vi "Tree.vi"   [LabVIEW 2016]
uses:
  subVIs/Add XY (single).vi
  subVIs/Add float (single).vi
  subVIs/Subtract float (single).vi
  subVIs/Multiply float (single).vi
  subVIs/Divide float (single).vi
  subVIs/Sort Ascending (multiple).vi
  subVIs/Decimate (multiple).vi
  subVIs/Add float (multiple).vi
  subVIs/Subtract float (multiple).vi
  subVIs/Multiply float (multiple).vi
  subVIs/Divide float (multiple).vi
  <vilib>/measure/maresamp.llb/Resample N Pairs of Arrays (single shot).vi
  subVIs/Derivative (multiple).vi
  subVIs/Derivative (single).vi
  subVIs/Sort Ascending (single).vi
  subVIs/Decimate (single).vi
  xy_utilities.lvlib
  <vilib>/measure/NI_MAPro.lvlib
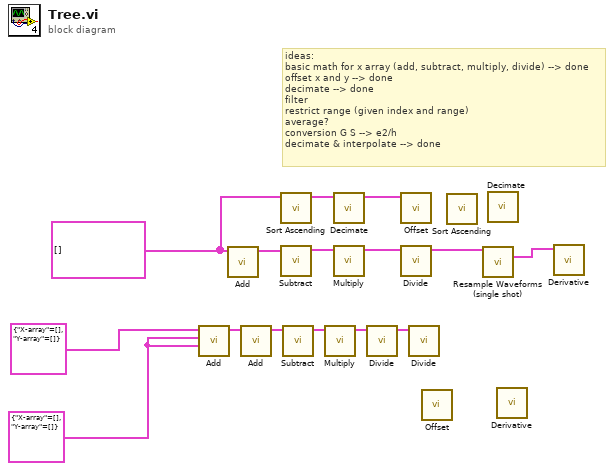
[diagram p0: block diagram]
diagram:
  w8 = cluster{"X-array":dbl[], "Y-array":dbl[]}[] [] ("Multiple XY-data in")
  w10 = cluster{"X-array":dbl[], "Y-array":dbl[]} {"X-array"=[], "Y-array"=[]} ("XY-data in")
  # "ideas:\nbasic math for x array (add, subtract, multiply, divide) --> done\noffset x and y --> done\ndecimate --> done\nfilter\nrestrict range (given index and range)\naverage?\nconversion G S --> e2/h\ndecimate & interpolate --> done"
  n1 = call-poly "Add.vi"("y XY-data in"=w10, "x XY-data in"=w10, "XY-data in"=cluster{"X-array":dbl[], "Y-array":dbl[]} {"X-array"=[], "Y-array"=[]}) -> ("XY-data out"=w5:cluster{"X-array":dbl[], "Y-array":dbl[]})  [unwired: 7 in, 1 out]
  n2 = call-poly "Add.vi"("Multiple XY-data in"=w8) -> ("Multiple XY-data out"=w13:cluster{"X-array":dbl[], "Y-array":dbl[]}[])  [unwired: 9 in, 1 out]
  n3 = call-poly "Add.vi"("XY-data in"=w5) -> ("XY-data out"=w4:cluster{"X-array":dbl[], "Y-array":dbl[]})  [unwired: 9 in, 1 out]
  n4 = call-poly "Sort Ascending.vi"("Multiple XY-data in"=w8) -> ("Multiple XY-data out"=w7:cluster{"X-array":dbl[], "Y-array":dbl[]}[])  [unwired: 9 in, 1 out]
  n5 = call-poly "Subtract.vi"("Multiple XY-data in"=w13) -> ("Multiple XY-data out"=w15:cluster{"X-array":dbl[], "Y-array":dbl[]}[])  [unwired: 9 in, 1 out]
  n6 = call-poly "Subtract.vi"("XY-data in"=w4) -> ("XY-data out"=w3:cluster{"X-array":dbl[], "Y-array":dbl[]})  [unwired: 9 in, 1 out]
  n7 = call-poly "Multiply.vi"("XY-data in"=w3) -> ("XY-data out"=w2:cluster{"X-array":dbl[], "Y-array":dbl[]})  [unwired: 9 in, 1 out]
  n8 = call-poly "Decimate.vi"("Multiple XY-data in"=w7) -> ("Multiple XY-data out"=w9:cluster{"X-array":dbl[], "Y-array":dbl[]}[])  [unwired: 9 in, 1 out]
  n9 = call-poly "Multiply.vi"("Multiple XY-data in"=w15) -> ("Multiple XY-data out"=w14:cluster{"X-array":dbl[], "Y-array":dbl[]}[])  [unwired: 9 in, 1 out]
  n10 = call-poly "Divide.vi"("XY-data in"=w2) -> ("XY-data out"=w1:cluster{"X-array":dbl[], "Y-array":dbl[]})  [unwired: 9 in, 1 out]
  n11 = call "Offset.vi"("Multiple XY-data in"=w9) -> ()  [unwired: 9 in, 2 out]
  n12 = call-poly "Divide.vi"("Multiple XY-data in"=w14) -> ("Multiple XY-data out"=w12:cluster{"X-array":dbl[], "Y-array":dbl[]}[])  [unwired: 9 in, 1 out]
  n13 = call-poly "Divide.vi"("XY-data in"=w1) -> ()  [unwired: 9 in, 2 out]
  n14 = call "Offset.vi"() -> ()  [unwired: 10 in, 2 out]
  n15 = call-poly "Sort Ascending.vi"() -> ()  [unwired: 10 in, 2 out]
  n16 = call-poly <vilib>:"Resample Waveforms (single shot).vi"("Multiple XY-data in"=w12) -> ("Multiple XY-data out"=w6:cluster{"X-array":dbl[], "Y-array":dbl[]}[])  [unwired: 10 in, 4 out]
  n17 = call-poly "Decimate.vi"() -> ()  [unwired: 10 in, 2 out]
  n18 = call-poly "Derivative.vi"() -> ()  [unwired: 10 in, 2 out]
  n19 = call-poly "Derivative.vi"("Multiple XY-data in"=w6) -> ()  [unwired: 9 in, 2 out]
